vi "Query with Scalar String Result.vi"(8 "error in (no error)":errorcluster, 10 "Query string":string, 11 "sqlite3 in":refnum<class "sqlite3.lvclass">) -> (0 "error out":errorcluster, 2 "Result":string, 3 "sqlite3 out":refnum<class "sqlite3.lvclass">)   [LabVIEW 2020, in "sqlite3.lvlib" / "sqlite3.lvclass"]
uses:
  sqlite3.lvclass
  sqlite3.lvclass/sqlite3.ctl
  40ca9895-98d3-4c11-8901-50168dec3d7c.vi
  sqlite/VIs/open v2.vi
  sqlite/VIs/close v2.vi
  sqlite/VIs/prepare v2.vi
  sqlite/VIs/step.vi
  sqlite/VIs/column count.vi
  db layer/compound/Resolve Result Type.vi
  40ca9895-98d3-4c11-8901-50168dec3d7c.vi/0244caef-bc9a-4150-a8ac-bf3d364b181c.vi
  40ca9895-98d3-4c11-8901-50168dec3d7c.vi/5568208c-18c9-421a-afbc-e39208249946.vi
  sqlite/VIs/finalize.vi
  sqlite/subvi/Error Converter (ErrCode or Status).vi
  sqlite/VIs/column type.vi
  sqlite/VIs/column text.vi
  sqlite/VIs/column bytes.vi
  sqlite/VIs/column blob.vi
  db layer/utilities/MoveBlock.vi
  sqlite/VIs/errstr.vi
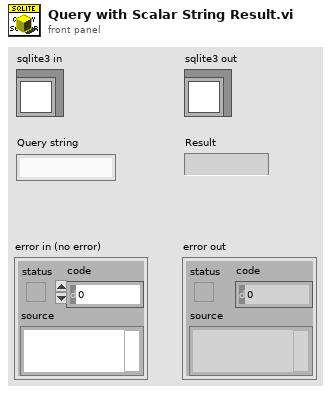
[diagram p1: front panel]
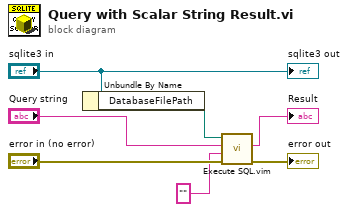
[diagram p0: block diagram]
diagram:
  n1 = Unbundle By Name("sqlite3 in") -> ("DatabaseFilePath"=w4:path)
  n2 = call "Execute SQL.vim"("error in (no error)"="error in (no error)", "desired return type(none)"="" ("Result"), "sql (string)"="Query string", "database in"=w4) -> ("error out"=→"error out":errorcluster, "Query Result"=→"Result":string)  [unwired: 6 in]
  "sqlite3 out" <- "sqlite3 in"
